vi "Correct_FFID_Bkgnd Header.vi"() -> (4 "Path":path)   [LabVIEW 2017]
panel:
  out "Channel Values Out":string[][](array[string])
  in  "Results file":path=path "Y:/Temporary Items/bkgnd_values.xls"
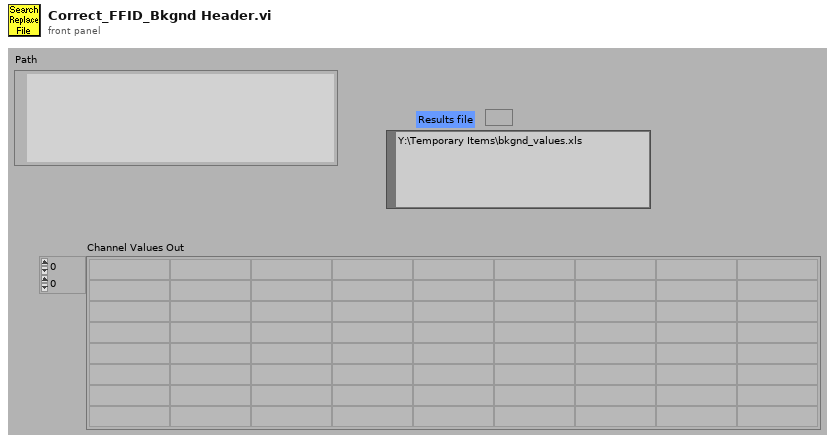
[diagram p1: front panel]
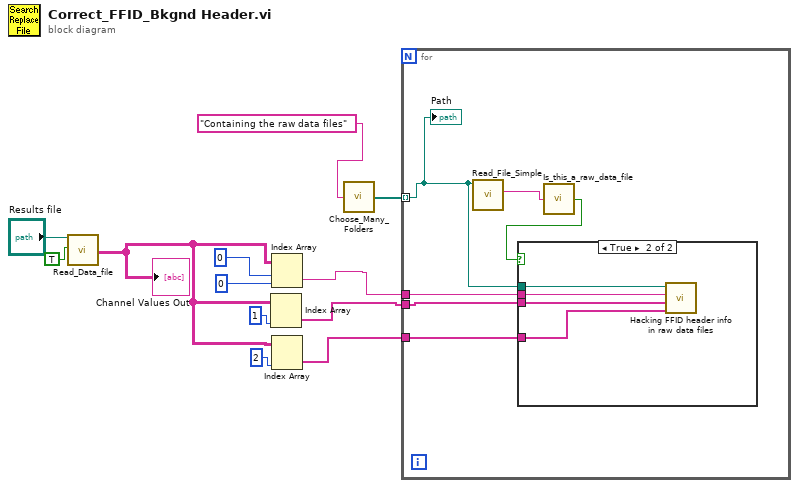
[diagram p0: block diagram]
diagram:
  n1 = call "Read_Data_file.vi"("Results file"="Results file", "Delete First Rows?"=TRUE) -> ("Channel Values Out"=w12:string[][])  [unwired: 5 in, 12 out]
  "Channel Values Out" <- w12
  n2 = Index Array(array=w12, index (col)=1 ("index (row)")) -> (element=w3:string[])  [unwired: 1 in]
  n3 = Index Array(array=w12, index (row)=0, index (col)=0 ("index (row)")) -> (element=w4:string)
  n4 = Index Array(array=w12, index (col)=2 ("index (row)")) -> (element=w2:string[])  [unwired: 1 in]
  n5 = call "Choose_Many_Folders.vi"("Purpose of choosing folder"="Containing the raw data files") -> ("Files"=w5:path[])
  n6 = for {
    tunnel: w5 -> [w13] mode=indexing
    tunnel: w4 -> [w18]
    tunnel: w3 -> [w17]
    tunnel: w2 -> [w16]
    n7 = call "Read_File_Simple.vi"("Filename"=w13) -> ("string"=w15:string)  [unwired: 4 in, 5 out]
    n8 = call "Is_this_a_raw_data_file.vi"("character string"=w15) -> ("Raw Dat File?"=w14:bool)  [unwired: 2 out]
    n9 = case shown="True" w14 {
      tunnel: w13 -> [_ w22]
      tunnel: w18 -> [_ w21]
      tunnel: w17 -> [_ w20]
      tunnel: w16 -> [_ w19]
      frame False {
      }
      frame True {
        n10 = call "Hacking FFID header info in raw data files.vi"("New Bkgnd Variance"=w19, "New Bkgnd Values"=w20, "Time"=w21, "file (use dialog)"=w22) -> ()  [unwired: 8 in]
      }
    }
    "Path" <- w13
  }
